vi "Brake.vi"(8 "Brake!":bool, 11 "error in (no error)":errorcluster) -> (3 "error out":errorcluster)   [LabVIEW 2016]
doc: "Inputs\nBrake\n\nOutputs\n-\n\nActivates the brake motor if the boolean input is true. It brakes for 3 seconds and then goes in reverse direction for 1 second to make sure the brake is not activated on the next run."
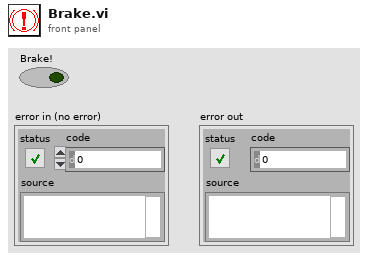
[diagram p1: front panel]
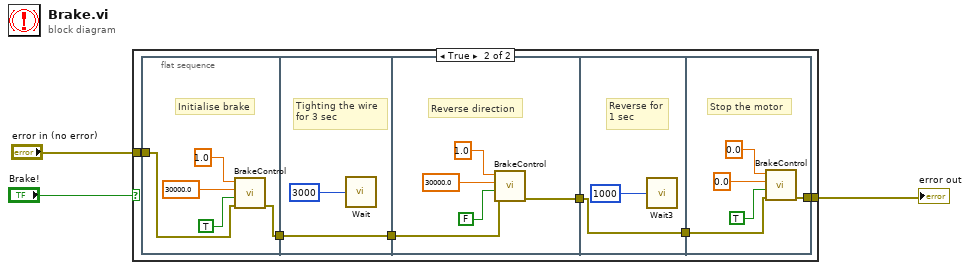
[diagram p0: block diagram]
diagram:
  n1 = case shown="True" "Brake!" {
    tunnel: "error in (no error)" -> [w4 w10]
    tunnel: [w4 w5] -> w3
    frame False {
    }
    frame True {
      n2 = flat-sequence {
        tunnel: w10 -> [w12]
        tunnel: [w11] -> w8
        tunnel: [w16] -> w9
        tunnel: w8 -> [w16]
        tunnel: [w19] -> w6
        tunnel: w9 -> [w18]
        tunnel: [w23] -> w7
        tunnel: w6 -> [w23]
        tunnel: w7 -> [w25]
        tunnel: [w26] -> w5
        frame #0 {
          # "Initialise brake"
          n3 = call "BrakeControl.vi"("error in (no error)"=w12, "Digital Input"=TRUE, "Frequency [Hz]"=30000.0, "Duty Cycle"=1.0) -> ("error out"=w11:errorcluster)  [unwired: 7 in]
        }
        frame #1 {
          # "Tighting the wire\nfor 3 sec"
          n4 = call "Wait"("Count(mSec)"=u32 3000) -> ()  [unwired: 1 out]
        }
        frame #2 {
          # "Reverse direction"
          n5 = call "BrakeControl.vi"("error in (no error)"=w18, "Digital Input"=FALSE, "Frequency [Hz]"=30000.0, "Duty Cycle"=1.0) -> ("error out"=w19:errorcluster)  [unwired: 7 in]
        }
        frame #3 {
          # "Reverse for\n1 sec"
          n6 = call "Wait3"("Count(mSec)"=u32 1000) -> ()  [unwired: 1 out]
        }
        frame #4 {
          # "Stop the motor"
          n7 = call "BrakeControl.vi"("error in (no error)"=w25, "Digital Input"=TRUE, "Frequency [Hz]"=0.0, "Duty Cycle"=0.0) -> ("error out"=w26:errorcluster)  [unwired: 7 in]
        }
      }
    }
  }
  "error out" <- w3
